vi "Arc test.vi"() -> ()   [LabVIEW 2015]
uses:
  <vilib>/myRIO/Instrument Drivers/Onboard IO/PWM/typedefs/PWM Reference.ctl
  <vilib>/myRIO/Common/Instrument Driver Framework/Utilities/typedefs/myRIO Generic Hardware Reference.ctl
  <vilib>/myRIO/Common/Instrument Driver Framework/Utilities/typedefs/Hardware Version Enum.ctl
  <vilib>/myRIO/Common/Instrument Driver Framework/Utilities/typedefs/myRIO v1.0 Reference.ctl
  <vilib>/myRIO/Common/Instrument Driver Framework/Utilities/typedefs/Generic FPGA Reference.ctl
  <vilib>/myRIO/Common/Instrument Driver Framework/myRIO v1.0/PWM/typedefs/PWM Channels Enum.ctl
  <vilib>/myRIO/Instrument Drivers/Onboard IO/PWM/typedefs/PWM Configuration.ctl
  <vilib>/userdefined/High Color/nirio_resource_hc.ctl
  <vilib>/myRIO/Common/Instrument Driver Framework/myRIO v1.0/PWM/vis/myRIO v1.1 Open PWM.vi
  <vilib>/myRIO/Common/Instrument Driver Framework/Utilities/vis/Validate Channels.vi
  <vilib>/myRIO/Common/Instrument Driver Framework/myRIO v1.0/PWM/vis/myRIO v1.0 Reserve PWM.vi
  <vilib>/myRIO/Instrument Drivers/Onboard IO/PWM/vis/Set Duty Cycle and Frequency.vi
  <vilib>/myRIO/Common/Instrument Driver Framework/myRIO v1.0/PWM/vis/myRIO v1.0 Build MUX Configuration PWM.vi
  <vilib>/myRIO/Common/Instrument Driver Framework/myRIO v1.0/Resource Manager/vis/myRIO v1.0 Reserve Channel List.vi
  <vilib>/myRIO/Common/Instrument Driver Framework/myRIO v1.0/Resource Manager/vis/myRIO v1.0 Create Configuration List.vi
  <vilib>/myRIO/Common/Instrument Driver Framework/myRIO v1.0/Resource Manager/vis/myRIO v1.0 Reserve Channel.vi
  <vilib>/myRIO/Common/Instrument Driver Framework/myRIO v1.0/Resource Manager/vis/myRIO v1.0 Unreserve Channel.vi
  <vilib>/myRIO/Common/Instrument Driver Framework/myRIO v1.0/Resource Manager/vis/myRIO v1.0 Build Mutex Name.vi
  <vilib>/Utility/VariantDataType/GetNumericInfo.vi
  <vilib>/Utility/error.llb/Error Cluster From Error Code.vi
  <vilib>/myRIO/Common/Instrument Driver Framework/myRIO v1.0/myRIO v1.1 Open.vi
  <vilib>/myRIO/Common/Instrument Driver Framework/Utilities/vis/IO Manager.vi
  <vilib>/myRIO/Common/Instrument Driver Framework/Utilities/vis/Configuration Manager.vi
  <vilib>/myRIO/Common/Instrument Driver Framework/myRIO v1.0/Resource Manager/vis/myRIO v1.0 Configure IO.vi
  <vilib>/myRIO/Common/Instrument Driver Framework/myRIO v1.0/myRIO v1.0 Close.vi
  <vilib>/myRIO/Common/Instrument Driver Framework/myRIO v1.0/PWM/vis/myRIO v1.0 Write PWM.vi
  <vilib>/myRIO/Instrument Drivers/Onboard IO/PWM/vis/myRIO PWM Open.xnode
  <vilib>/myRIO/Instrument Drivers/Onboard IO/PWM/PWM.lvlib
panel:
  in  "L Duty Cycle":dbl=0.63 format="%#_13g"
  in  "R Duty Cycle":dbl=0.55 format="%#_13g"
  in  "stop":bool
  in  "Boolean":bool
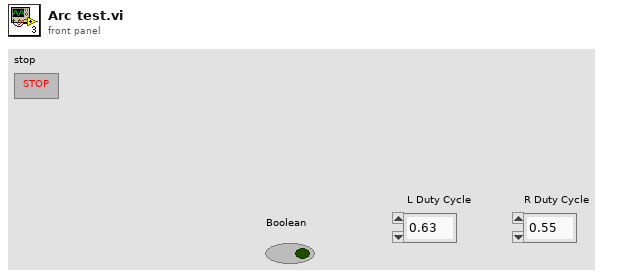
[diagram p1: front panel]
types:
  T1 = typedef "PWM.lvlib/PWM Reference.ctl" = cluster{"myRIO Reference":T2, "PWM Channels Enum":T6, "PWM Configuration":T7}
  T2 = typedef "myRIO Generic Hardware Reference.ctl" = cluster{"myRIO Model":T3, "myRIO Hardware Reference":T4}
  T3 = typedef "Hardware Version Enum.ctl" = enum16{"Unknown", "myRIO-1900", "myRIO-1950", "roboRIO"}
  T4 = typedef "myRIO v1.0 Reference.ctl" = cluster{"Generic FPGA Reference":T5, "Allow multiple opens":bool}
  T5 = typedef "Generic FPGA Reference.ctl" = refnum<k20>
  T6 = typedef "PWM Channels Enum.ctl" = enum16{"Not Connected", "C/PWM0", "C/PWM1", "A/PWM0", "A/PWM1", "A/PWM2", "B/PWM0", "B/PWM1", "B/PWM2", "PWM/PWM0", "PWM/PWM1", "PWM/PWM2", "PWM/PWM3", "PWM/PWM4", "PWM/PWM5", "PWM/PWM6", "PWM/PWM7", "PWM/PWM8", "PWM/PWM9"}
  T7 = typedef "PWM.lvlib/PWM Configuration.ctl" = cluster{"Frequency":dbl, "Duty Cycle":dbl}
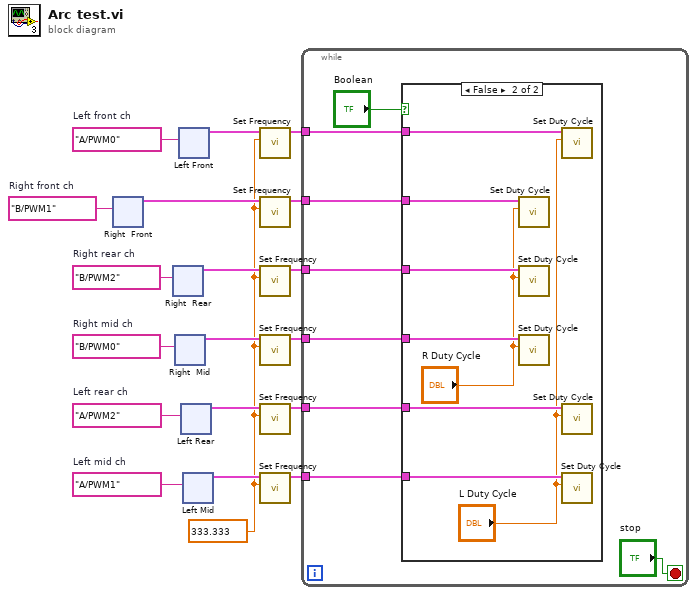
[diagram p0: block diagram]
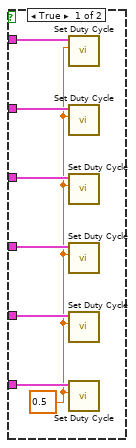
[diagram p2: hidden frame]
diagram:
  w1 = 333.333 ("Frequency [Hz]")
  w14 = tag "B/PWM2"  # Right rear ch
  w15 = tag "B/PWM0"  # Right mid ch
  w16 = tag "B/PWM1"  # Right front ch
  w17 = tag "A/PWM2"  # Left rear ch
  w18 = tag "A/PWM1"  # Left mid ch
  w19 = tag "A/PWM0"  # Left front ch
  n1 = xnode "Right  Front"("Channel Name"=w16) -> ("PWM Ref Out"=w10:T1)  [unwired: 2 in, 1 out]
  n2 = xnode "Right  Rear"("Channel Name"=w14) -> ("PWM Ref Out"=w8:T1)  [unwired: 2 in, 1 out]
  n3 = xnode "Right  Mid"("Channel Name"=w15) -> ("PWM Ref Out"=w9:T1)  [unwired: 2 in, 1 out]
  n4 = xnode "Left Front"("Channel Name"=w19) -> ("PWM Ref Out"=w13:T1)  [unwired: 2 in, 1 out]
  n5 = xnode "Left Rear"("Channel Name"=w17) -> ("PWM Ref Out"=w11:T1)  [unwired: 2 in, 1 out]
  n6 = xnode "Left Mid"("Channel Name"=w18) -> ("PWM Ref Out"=w12:T1)  [unwired: 2 in, 1 out]
  n7 = call <vilib>:"Set Frequency.vi"("Frequency [Hz]"=w1, "PWM Ref In"=w13) -> ("PWM Ref Out"=w7:T1)  [unwired: 7 in, 1 out]
  n8 = call <vilib>:"Set Frequency.vi"("Frequency [Hz]"=w1, "PWM Ref In"=w10) -> ("PWM Ref Out"=w4:T1)  [unwired: 7 in, 1 out]
  n9 = call <vilib>:"Set Frequency.vi"("Frequency [Hz]"=w1, "PWM Ref In"=w8) -> ("PWM Ref Out"=w6:T1)  [unwired: 7 in, 1 out]
  n10 = call <vilib>:"Set Frequency.vi"("Frequency [Hz]"=w1, "PWM Ref In"=w9) -> ("PWM Ref Out"=w5:T1)  [unwired: 7 in, 1 out]
  n11 = call <vilib>:"Set Frequency.vi"("Frequency [Hz]"=w1, "PWM Ref In"=w11) -> ("PWM Ref Out"=w3:T1)  [unwired: 7 in, 1 out]
  n12 = call <vilib>:"Set Frequency.vi"("Frequency [Hz]"=w1, "PWM Ref In"=w12) -> ("PWM Ref Out"=w2:T1)  [unwired: 7 in, 1 out]
  n13 = while {
    tunnel: w7 -> [w27]
    tunnel: w6 -> [w26]
    tunnel: w5 -> [w25]
    tunnel: w4 -> [w24]
    tunnel: w3 -> [w23]
    tunnel: w2 -> [w22]
    stop <- "stop" stop-if-true
    n14 = case shown="False" "Boolean" {
      tunnel: w27 -> [w34 w42]
      tunnel: w26 -> [w33 w41]
      tunnel: w25 -> [w32 w40]
      tunnel: w24 -> [w31 w39]
      tunnel: w23 -> [w30 w38]
      tunnel: w22 -> [w29 w37]
      frame True {
        w28 = 0.5 ("Duty Cycle")
        n15 = call <vilib>:"Set Duty Cycle.vi"("Duty Cycle"=w28, "PWM Ref In"=w34) -> ()  [unwired: 7 in, 2 out]
        n16 = call <vilib>:"Set Duty Cycle.vi"("Duty Cycle"=w28, "PWM Ref In"=w31) -> ()  [unwired: 7 in, 2 out]
        n17 = call <vilib>:"Set Duty Cycle.vi"("Duty Cycle"=w28, "PWM Ref In"=w33) -> ()  [unwired: 7 in, 2 out]
        n18 = call <vilib>:"Set Duty Cycle.vi"("Duty Cycle"=w28, "PWM Ref In"=w32) -> ()  [unwired: 7 in, 2 out]
        n19 = call <vilib>:"Set Duty Cycle.vi"("Duty Cycle"=w28, "PWM Ref In"=w30) -> ()  [unwired: 7 in, 2 out]
        n20 = call <vilib>:"Set Duty Cycle.vi"("Duty Cycle"=w28, "PWM Ref In"=w29) -> ()  [unwired: 7 in, 2 out]
      }
      frame False {
        n21 = call <vilib>:"Set Duty Cycle.vi"("Duty Cycle"="R Duty Cycle", "PWM Ref In"=w39) -> ()  [unwired: 7 in, 2 out]
        n22 = call <vilib>:"Set Duty Cycle.vi"("Duty Cycle"="R Duty Cycle", "PWM Ref In"=w41) -> ()  [unwired: 7 in, 2 out]
        n23 = call <vilib>:"Set Duty Cycle.vi"("Duty Cycle"="R Duty Cycle", "PWM Ref In"=w40) -> ()  [unwired: 7 in, 2 out]
        n24 = call <vilib>:"Set Duty Cycle.vi"("Duty Cycle"="L Duty Cycle", "PWM Ref In"=w42) -> ()  [unwired: 7 in, 2 out]
        n25 = call <vilib>:"Set Duty Cycle.vi"("Duty Cycle"="L Duty Cycle", "PWM Ref In"=w38) -> ()  [unwired: 7 in, 2 out]
        n26 = call <vilib>:"Set Duty Cycle.vi"("Duty Cycle"="L Duty Cycle", "PWM Ref In"=w37) -> ()  [unwired: 7 in, 2 out]
      }
    }
  }
